vi "DT_Scope.vi"() -> ()   [LabVIEW 2012]
doc: "The DtAinContinuous example demonstrates how to continuously acquire data from an analog input channel. This example runs continuously until either the Stop button is pressed or an error occurs."
uses:
  <userlib>/LV-Link3/PolySubVIs/DtCreateAinChan.vi
  <userlib>/LV-Link3/PolySubVIs/DtOLTimingSetInput.vi
  <userlib>/LV-Link3/PolySubVIs/DtOLReadMultiple2D.vi
  <vilib>/Analysis/baseanly.llb/Mean (DBL).vi
  <vilib>/Analysis/NI_AALBase.lvlib
panel:
  out "Averages":dbl[](array[numeric])
  in  "Ch Numbers":i64[](array[numeric])=[0]
  out "Acquired Data":dbl[][](graph)
  in  "Samples Per Channel":dbl=1000.0
  in  "Sample Rate":dbl=10000.0
  in  "?":bool
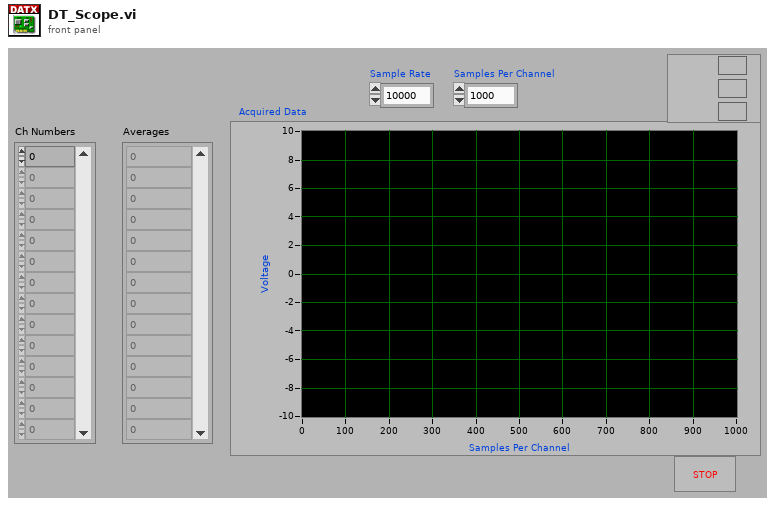
[diagram p1: front panel]
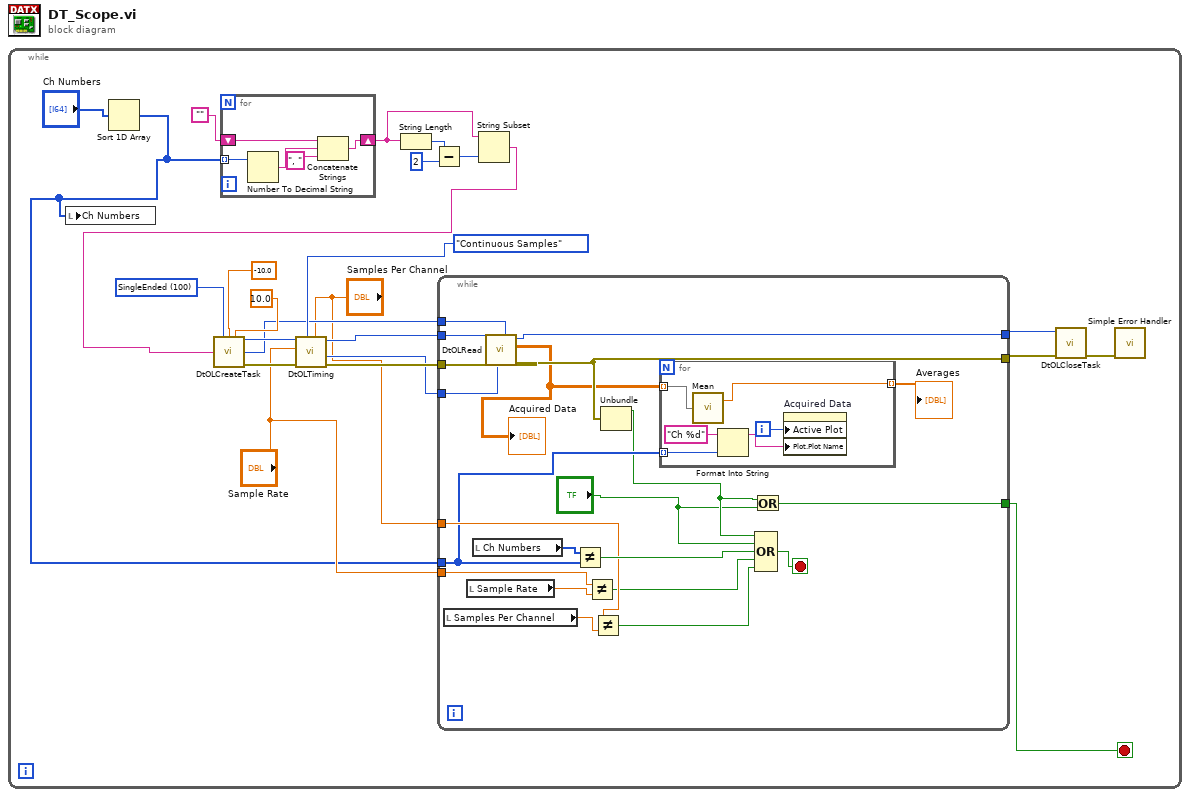
[diagram p0: block diagram]
diagram:
  n1 = while {
    stop <- w3 stop-if-true
    w17 = 100 items=["SingleEnded"=100, "Differential"=101] ("Channel Type")
    n2 = Sort 1D Array(array="Ch Numbers") -> (sorted array=w1:i64[])
    n3 = local write "Ch Numbers"(w1) -> ()
    n4 = for {
      tunnel: w1 -> [w29] mode=indexing
      shift-right: [w25] -> w8
      shift-left: "" -> [w26]
      n5 = Number To Decimal String(number=w29) -> (decimal integer string=w28:string)  [unwired: 1 in]
      n6 = Concatenate Strings(w26, w28, ", " ("string")) -> (w25:string)
    }
    n7 = String Length(string=w8) -> (length=w7:i32)
    n8 = Subtract(x=w7, y=2) -> (x-y=w5:i32)
    n9 = String Subset(string=w8, length (rest)=w5) -> (substring=w4:string)  [unwired: 1 in]
    n10 = call-poly <userlib>:"DtOLCreateTask.vi"("Channel Type"=w17, "Range Min"=-10.0, "Range Max"=10.0, "Channel"=w4) -> ("Task out"=w15:i32, "Actual Number of Channels"=w13:u32, "error out"=w24:errorcluster)  [unwired: 9 in]
    n11 = call-poly <userlib>:"DtOLTiming.vi"("Samples Per Channel"="Samples Per Channel", "Sample Mode"=enum16{"Finite Samples", "Continuous Samples"}."Continuous Samples", "error in (no error)"=w24, "Sample Freq (Hz)"="Sample Rate", "Task in"=w15) -> ("error out"=w18:errorcluster, "Buffer Size"=w12:u32, "Task out"=w19:i32)  [unwired: 3 in, 1 out]
    n12 = while {
      tunnel: w18 -> [w50]
      tunnel: [w49] -> w21
      tunnel: [w48] -> w20
      tunnel: w19 -> [w47]
      tunnel: w13 -> [w46]
      tunnel: w12 -> [w45]
      tunnel: w1 -> [w33]
      tunnel: "Sample Rate" -> [w40]
      tunnel: "Samples Per Channel" -> [w39]
      tunnel: [w30] -> w3
      stop <- w36 stop-if-true
      n13 = local read "Samples Per Channel"() -> (w41:dbl)
      n14 = local read "Sample Rate"() -> (w42:dbl)
      n15 = local read "Ch Numbers"() -> (w44:i64[])
      n16 = call-poly <userlib>:"DtOLRead.vi"("Number Chan to Read"=w46, "Buffer size"=w45, "error in (no error)"=w50, "Task in"=w47) -> ("error out"=w48:errorcluster, "2D Data out"=w35:dbl[][], "Task out"=w49:i32)  [unwired: 3 in, 2 out]
      "Acquired Data" <- w35
      n17 = Not Equal?(x=w44, y=w33) -> (x != y?=w43:bool)
      n18 = Not Equal?(x=w40, y=w42) -> (x != y?=w38:bool)
      n19 = Not Equal?(x=w39, y=w41) -> (x != y?=w37:bool)
      n20 = Unbundle(w48) -> ("status"=w32:bool)  [unwired: 2 out]
      n21 = for {
        tunnel: w35 -> [w56] mode=indexing
        tunnel: [w55] -> w34 mode=indexing
        tunnel: w33 -> [w53] mode=indexing
        i -> [w54]
        n22 = call-poly <vilib>:"Mean.vi"("X"=w56) -> ("mean"=w55:dbl)  [unwired: 1 out]
        n23 = Format Into String(format string="Ch %d", w53) -> (resulting string=w51:string)  [unwired: 2 in, 1 out]
        n24 = property on="Acquired Data" class="WFGraph (strict)"("Active Plot"=w54, "Plot.Plot Name"=w51) -> ()  [unwired: 2 in, 2 out]
      }
      "Averages" <- w34
      n25 = Or(x=w32, y="?") -> (x .or. y?=w30:bool)
      n26 = Compound Arithmetic op=OR(w32, "?", w43, w38, w37) -> (w36:bool)
    }
    n27 = call <userlib>:"DtOLCloseTask.vi"("Error in"=w20, "Task in"=w21) -> ("Error Out"=w22:errorcluster)  [unwired: 9 in]
    n28 = call <vilib>:"Simple Error Handler.vi"("error in (no error)"=w22) -> ()  [unwired: 4 in, 5 out]
  }
